vi "Scan_Update.vi"(8 "Error In":errorcluster caption="错误输入", 11 "键盘设备":refnum<k1> caption="设备ID输出") -> (0 "Error Out":errorcluster caption="错误输出", 1 "偏振光角度":dbl, 2 "Y轴位置":dbl, 3 "X轴位置":dbl)   [LabVIEW 2020]
uses:
  CH375/Global_CH375.vi
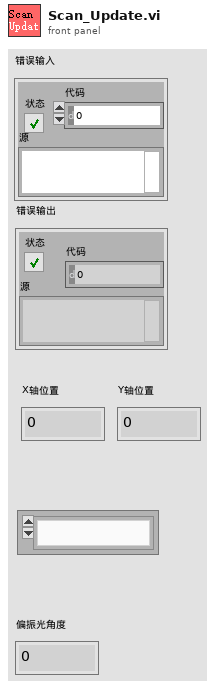
[diagram p1: front panel]
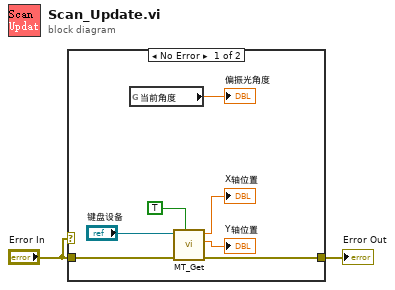
[diagram p0: block diagram]
diagram:
  n1 = case shown="No Error" "Error In" {
    tunnel: "Error In" -> [w9 w10]
    tunnel: [w8 w10] -> w1
    frame No Error {
      n2 = global read "Global_CH375.vi" "当前角度"() -> (→"偏振光角度":dbl)
      n3 = call "MT_Get.vi"("手动操作(False)"=TRUE, "Error In"=w9, "键盘设备输入"="键盘设备") -> ("Error Out"=w8:errorcluster, "Y轴位置"=→"Y轴位置":dbl, "X轴位置"=→"X轴位置":dbl)  [unwired: 4 in, 2 out]
    }
    frame Error {
    }
  }
  "Error Out" <- w1
